vi "SNRNew.vi"(11 "Constellation":cdb[](array[numeric])) -> (1 "sum 2":dbl, 2 "sum 3":dbl, 3 "sum 1":dbl, 4 "SNR":dbl)   [LabVIEW 2018]
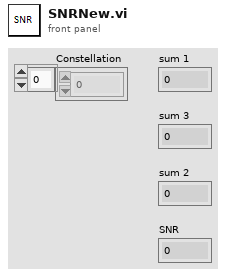
[diagram p1: front panel]
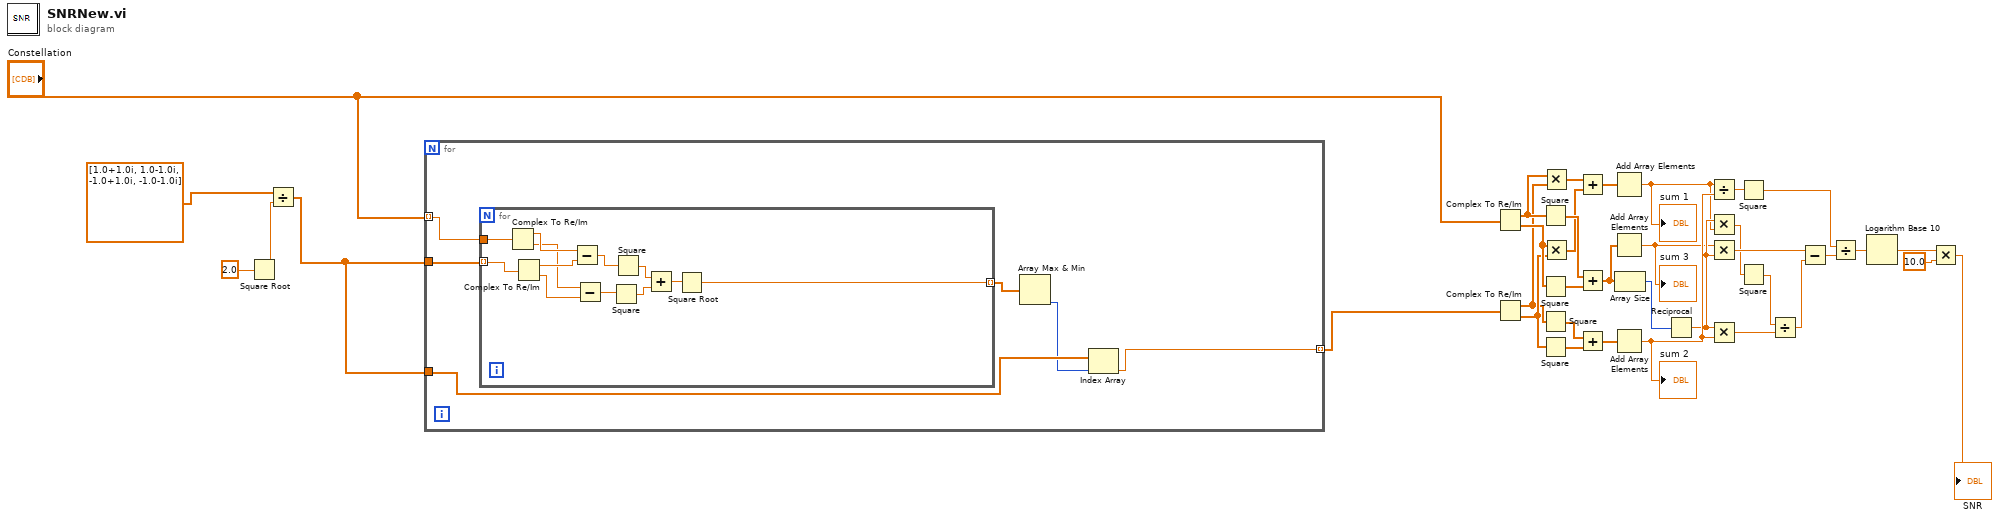
[diagram p0: block diagram]
diagram:
  n1 = Square Root(x=2.0) -> (sqrt(x)=w3:dbl)
  n2 = Divide(x=cdb[] [1.0+1.0i, 1.0-1.0i, -1.0+1.0i, -1.0-1.0i], y=w3) -> (x/y=w4:cdb[])
  n3 = for {
    tunnel: "Constellation" -> [w41] mode=indexing
    tunnel: w4 -> [w42]
    tunnel: w4 -> [w39]
    tunnel: [w37] -> w36 mode=indexing
    n4 = for {
      tunnel: w42 -> [w54] mode=indexing
      tunnel: w41 -> [w53]
      tunnel: [w43] -> w40 mode=indexing
      n5 = Complex To Re/Im(x + iy=w53) -> (x=w52:dbl, y=w50:dbl)
      n6 = Complex To Re/Im(x + iy=w54) -> (x=w51:dbl, y=w49:dbl)
      n7 = Subtract(x=w52, y=w51) -> (x-y=w48:dbl)
      n8 = Subtract(x=w50, y=w49) -> (x-y=w47:dbl)
      n9 = Square(x=w47) -> (x^2=w46:dbl)
      n10 = Square(x=w48) -> (x^2=w45:dbl)
      n11 = Add(x=w45, y=w46) -> (x+y=w44:dbl)
      n12 = Square Root(x=w44) -> (sqrt(x)=w43:dbl)
    }
    n13 = Array Max & Min(array=w40) -> (min index (indices)=w38:i32)  [unwired: 3 out]
    n14 = Index Array(array=w39, index=w38) -> (element=w37:cdb)
  }
  n15 = Complex To Re/Im(x + iy="Constellation") -> (x=w15:dbl[], y=w16:dbl[])
  n16 = Complex To Re/Im(x + iy=w36) -> (x=w8:dbl[], y=w9:dbl[])
  n17 = Square(x=w15) -> (x^2=w13:dbl[])
  n18 = Square(x=w16) -> (x^2=w14:dbl[])
  n19 = Square(x=w8) -> (x^2=w10:dbl[])
  n20 = Square(x=w9) -> (x^2=w11:dbl[])
  n21 = Multiply(x=w15, y=w8) -> (x*y=w5:dbl[])
  n22 = Multiply(x=w16, y=w9) -> (x*y=w6:dbl[])
  n23 = Add(x=w5, y=w6) -> (x+y=w7:dbl[])
  n24 = Add(x=w13, y=w14) -> (x+y=w17:dbl[])
  n25 = Add(x=w10, y=w11) -> (x+y=w12:dbl[])
  n26 = Add Array Elements(numeric array=w7) -> (sum=w21:dbl)
  "sum 1" <- w21
  n27 = Add Array Elements(numeric array=w17) -> (sum=w20:dbl)
  "sum 3" <- w20
  n28 = Add Array Elements(numeric array=w12) -> (sum=w25:dbl)
  "sum 2" <- w25
  n29 = Array Size(array=w17) -> (size(s)=w18:i32)
  n30 = Reciprocal(x=w18) -> (1/x=w24:dbl)
  n31 = Divide(x=w21, y=w25) -> (x/y=w19:dbl)
  n32 = Multiply(x=w24, y=w21) -> (x*y=w22:dbl)
  n33 = Multiply(x=w20, y=w24) -> (x*y=w27:dbl)
  n34 = Multiply(x=w24, y=w25) -> (x*y=w26:dbl)
  n35 = Square(x=w19) -> (x^2=w30:dbl)
  n36 = Square(x=w22) -> (x^2=w23:dbl)
  n37 = Divide(x=w23, y=w26) -> (x/y=w28:dbl)
  n38 = Subtract(x=w27, y=w28) -> (x-y=w29:dbl)
  n39 = Divide(x=w30, y=w29) -> (x/y=w31:dbl)
  n40 = Logarithm Base 10(1:w31) -> (0:w32:dbl)
  n41 = Multiply(x=w32, y=10.0) -> (x*y=→"SNR":dbl)
